vi "ODBC_test.vi"() -> ()   [LabVIEW 2011]
panel:
  out "concatenated string":string
  out "Error":bool
  in  "Notes":string="this is a test"
  in  "Operator Name":string="PA"
  in  "Database File":path=path "C:/MOCVD/MOCVD_Growths_test.accdb"
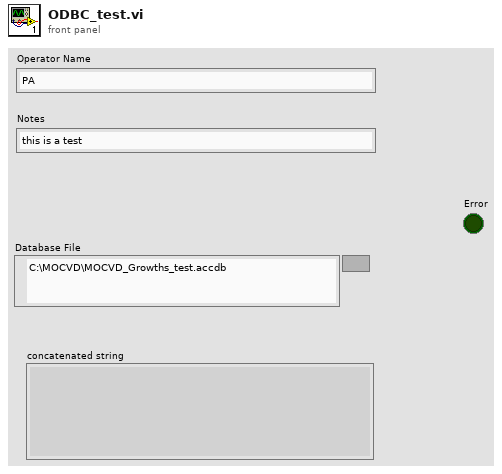
[diagram p1: front panel]
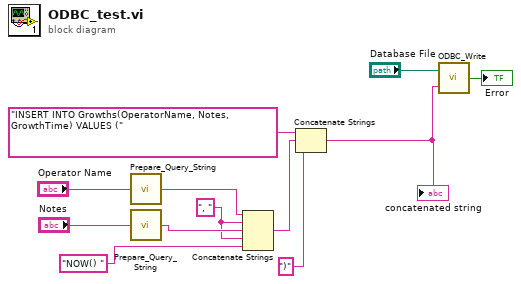
[diagram p0: block diagram]
diagram:
  w3 = ", " ("string")
  n1 = call "Prepare_Query_String.vi"("Input String"="Operator Name") -> ("Output String"=w8:string)
  n2 = call "Prepare_Query_String.vi"("Input String"="Notes") -> ("Output String"=w7:string)
  n3 = Concatenate Strings(w8, w3, w7, w3, "NOW() " ("string")) -> (w6:string)
  n4 = Concatenate Strings("INSERT INTO Growths(OperatorName, Notes, GrowthTime) VALUES (" ("string"), w6, ")" ("string")) -> (w2:string)
  "concatenated string" <- w2
  n5 = call "ODBC_Write.vi"("Query"=w2, "Database File"="Database File") -> ("Error"=→"Error":bool)
